vi "BOX_TO_BOX(SubVI).vi"(1 "Bounding Box 2":cluster{"x":sgl, "y":sgl}[](array[cluster]), 2 "Bounding Box 1":cluster{"x":sgl, "y":sgl}[](array[cluster])) -> (0 "Bounding Box Out":cluster{"x":sgl, "y":sgl}[](array[cluster]))   [LabVIEW 2011]
doc: "Recuadra a partir de dos recuadros, como hace el rect to rect de openG, pero apartir de las Bounding Box."
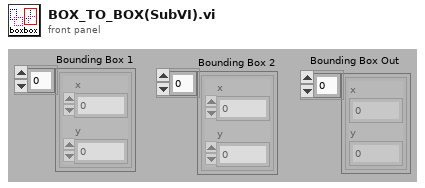
[diagram p1: front panel]
types:
  T1 = cluster{"left":i16, "top":i16, "right":i16, "bottom":i16}
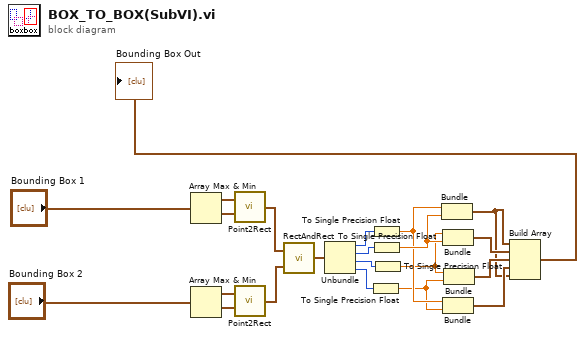
[diagram p0: block diagram]
diagram:
  n1 = Array Max & Min(array="Bounding Box 1") -> (max value=w2:cluster{"x":sgl, "y":sgl}, min value=w3:cluster{"x":sgl, "y":sgl})  [unwired: 2 out]
  n2 = Array Max & Min(array="Bounding Box 2") -> (max value=w4:cluster{"x":sgl, "y":sgl}, min value=w5:cluster{"x":sgl, "y":sgl})  [unwired: 2 out]
  n3 = call "Point2Rect.vi"("point b"=w3, "point a"=w2) -> ("rect"=w7:T1)
  n4 = call "Point2Rect.vi"("point b"=w5, "point a"=w4) -> ("rect"=w8:T1)
  n5 = call "RectAndRect.vi"("rect b"=w8, "rect a"=w7) -> ("union rect"=w21:T1)
  n6 = Unbundle(w21) -> ("left"=w18:i16, "top"=w19:i16, "right"=w20:i16, "bottom"=w17:i16)
  n7 = To Single Precision Float(number=w17) -> (single precision float=w14:sgl)
  n8 = To Single Precision Float(number=w18) -> (single precision float=w15:sgl)
  n9 = To Single Precision Float(number=w19) -> (single precision float=w16:sgl)
  n10 = To Single Precision Float(number=w20) -> (single precision float=w13:sgl)
  n11 = Bundle(w15, w16) -> (w9:cluster{sgl, sgl})  [unwired: 1 out]
  n12 = Bundle(w13, w16) -> (w12:cluster{sgl, sgl})  [unwired: 1 out]
  n13 = Bundle(w15, w14) -> (w10:cluster{sgl, sgl})  [unwired: 1 out]
  n14 = Bundle(w13, w14) -> (w11:cluster{sgl, sgl})  [unwired: 1 out]
  n15 = Build Array(w9, w12, w11, w10, w9) -> (→"Bounding Box Out":cluster{sgl, sgl}[])
